vi "24C and 4G Read (SubVI).vi"(11 "Instrument":T4={"335 Resource"="", "Input (0:A)"=0, "Instrument Type"=enum."PPMS", "quantum design"=refnum, "Heater Output (1:1)"=0, "semaphore"=refnum, "TCP master instance"=refnum, "335 Status"=refnum, "M24C Resource"="GPIB0::24::INSTR", "4G supply"="GPIB0::24::INSTR", "Temp Status 24C"=refnum, "Temp"=refnum, "9T信号"=refnum, "limit"={"Field limit"=0.0, "Field rate limit"=0.0, "Temp limit"=0.0, "Temp low limit"=0.0, "Temp rate limit "=0.0}, "4g supply status"=refnum, "vi路径"=""} {"Input (0:A)" items=["A", "B"]; "Heater Output (1:1)" items=["1"=1, "2"=2]}) -> (0 "field status":T1=enum."Stable", 1 "field(Oe)":dbl, 2 "输出簇":T3 {"Loop1 Output (%)" format="%.2f"; "Loop2 Output (%)" format="%.2f"}, 3 "下拉列表":T2 items=["Unknow", "Stable", "Following Warm", "Following Cold", "Unfollowing"])   [LabVIEW 2019, in "9T cmag.lvlib"]
uses:
  9T cmag.lvlib
  ctl/Instrument.ctl
  <vilib>/NI/Modbus Library/API/Master/Modbus Master.lvclass
  ctl/Instrument Type.ctl
  lib/QDInstrument.dll
  ctl/335 state.ctl
  ctl/limit.ctl
  ctl/9T mag field stauts.ctl
  User lib.lvlib
panel:
  out "x-y 2":dbl
  out "x-y":dbl
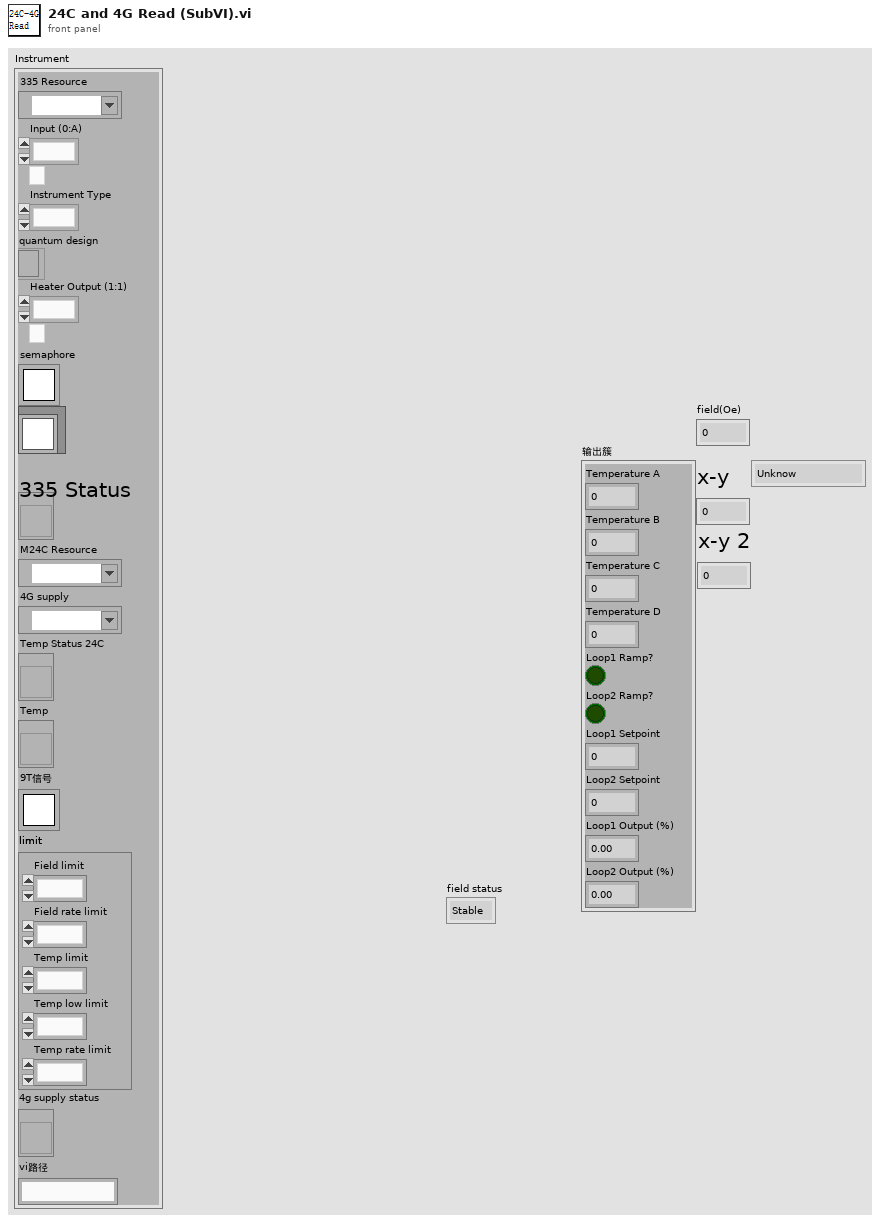
[diagram p1: front panel]
types:
  T1 = typedef "9T mag field stauts.ctl" = enum16{"unknow", "Stable", "Sweep up", "Sweep down", "Sweep to zero", "Pause"}
  T2 = typedef "335 state.ctl" = u16
  T3 = cluster{"Temperature A":dbl, "Temperature B":dbl, "Temperature C":dbl, "Temperature D":dbl, "Loop1 Ramp?":bool, "Loop2 Ramp?":bool, "Loop1 Setpoint":dbl, "Loop2 Setpoint":dbl, "Output Pwr (%)":dbl, "Output Pwr (%)":dbl}
  T4 = typedef "Instrument.ctl" = cluster{"335 Resource":refnum<visa-resource-name>, "Input (0:A)":u16, "Instrument Type":T5, "quantum design":refnum<k24>, "Heater Output (1:1)":u16, "semaphore":T6, "TCP master instance":refnum<class "Modbus Master.lvclass">, "335 Status":refnum<vi>, "M24C Resource":refnum<visa-resource-name>, "4G supply":refnum<visa-resource-name>, "Temp Status 24C":refnum<vi>, "Temp":refnum<vi>, "9T信号":T6, "limit":T7, "4g supply status":refnum<vi>, "vi路径":string}
  T5 = typedef "Instrument Type.ctl" = enum16{"PPMS", "VersaLab", "DynaCool", "SVSM", "PPMS-Rotate", "Lakeshore335", "9T mag"}
  T6 = typedef "Semaphore RefNum" = refnum<k1>
  T7 = typedef "limit.ctl" = cluster{"Field limit":dbl, "Field rate limit":dbl, "Temp limit":dbl, "Temp low limit":dbl, "Temp rate limit ":dbl}
  T8 = cluster{"Temperature":dbl, "Temperature":dbl, "Temperature":dbl, "Temperature":dbl, "x = y?":bool, "x = y?":bool, "数字":dbl, "数字":dbl, "Output Pwr (%)":dbl, "Output Pwr (%)":dbl}
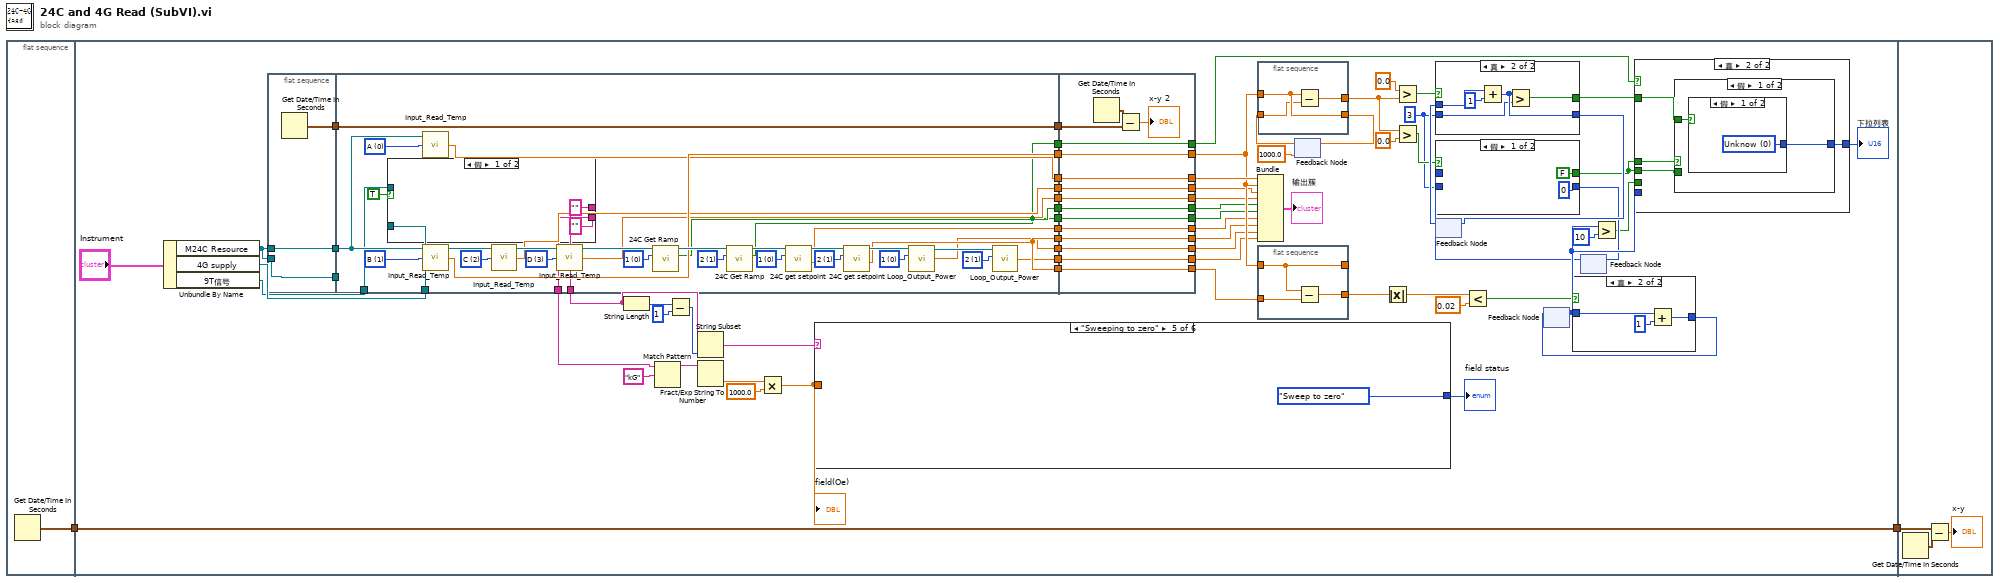
[diagram p0: block diagram]
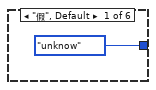
[diagram p2: hidden frame]
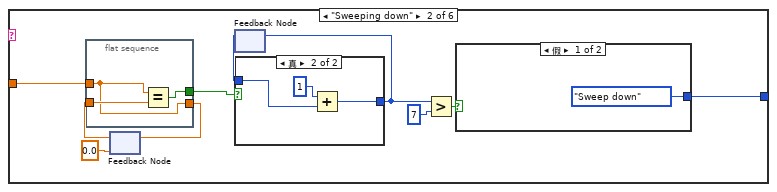
[diagram p3: hidden frame]
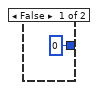
[diagram p4: hidden frame]
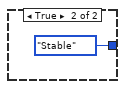
[diagram p5: hidden frame]
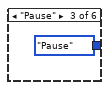
[diagram p6: hidden frame]
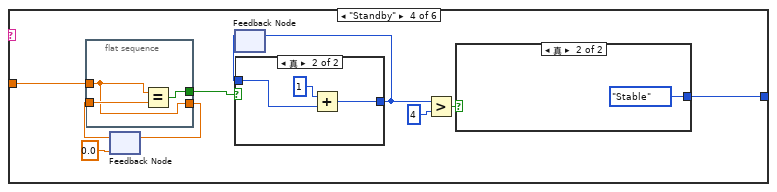
[diagram p7: hidden frame]
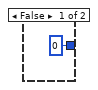
[diagram p8: hidden frame]
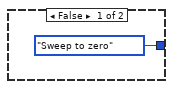
[diagram p9: hidden frame]
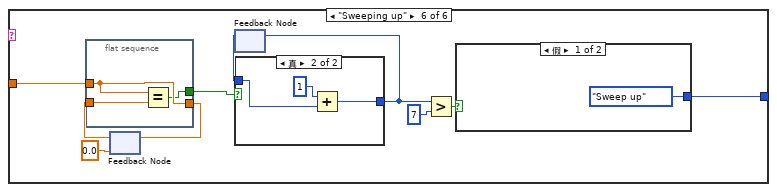
[diagram p10: hidden frame]
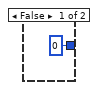
[diagram p11: hidden frame]
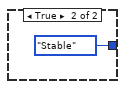
[diagram p12: hidden frame]
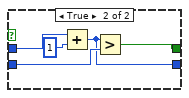
[diagram p13: hidden frame]
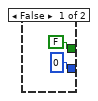
[diagram p14: hidden frame]
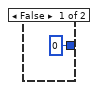
[diagram p15: hidden frame]
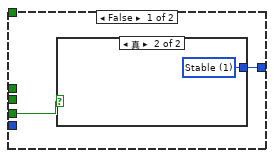
[diagram p16: hidden frame]
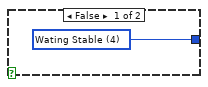
[diagram p17: hidden frame]
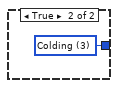
[diagram p18: hidden frame]
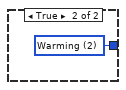
[diagram p19: hidden frame]
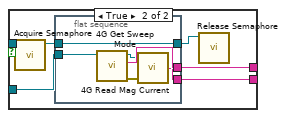
[diagram p20: hidden frame]
diagram:
  n1 = flat-sequence {
    tunnel: [w3] -> w2
    tunnel: w2 -> [w34]
    tunnel: [w34] -> w1
    tunnel: w1 -> [w240]
    frame #0 {
      n2 = Get Date/Time In Seconds() -> (seconds since 1Jan1904=w3:timestamp)
    }
    frame #1 {
      w57 = 3 ("y")
      n3 = Unbundle By Name("Instrument") -> ("M24C Resource"=w56:refnum<visa-resource-name>, "4G supply"=w35:refnum<visa-resource-name>, "9T信号"=w16:T6)
      n4 = flat-sequence {
        tunnel: w56 -> [w172]
        tunnel: w56 -> [w173]
        tunnel: [w173] -> w33
        tunnel: [w172] -> w32
        tunnel: [w171] -> w19
        tunnel: [w176] -> w4
        tunnel: [w180] -> w7
        tunnel: w35 -> [w179]
        tunnel: w33 -> [_]
        tunnel: w32 -> [w178]
        tunnel: [w195] -> w31
        tunnel: [w185] -> w30
        tunnel: [w183] -> w29
        tunnel: [w189] -> w28
        tunnel: [w188] -> w27
        tunnel: [w187] -> w26
        tunnel: [w186] -> w25
        tunnel: [w185] -> w24
        tunnel: [w184] -> w23
        tunnel: [w183] -> w22
        tunnel: [w182] -> w21
        tunnel: [w181] -> w20
        tunnel: w19 -> [w177]
        tunnel: [w177] -> w18
        tunnel: w16 -> [w175]
        tunnel: [w226] -> w37
        tunnel: [w227] -> w38
        tunnel: [w228] -> w39
        tunnel: [w229] -> w40
        tunnel: [w230] -> w41
        tunnel: [w231] -> w42
        tunnel: [w232] -> w43
        tunnel: [w233] -> w44
        tunnel: [w234] -> w46
        tunnel: [w235] -> w52
        tunnel: [w236] -> w53
        tunnel: [w237] -> w45
        tunnel: w31 -> [w237]
        tunnel: w30 -> [w236]
        tunnel: w29 -> [w235]
        tunnel: w28 -> [w234]
        tunnel: w27 -> [w233]
        tunnel: w26 -> [w232]
        tunnel: w25 -> [w231]
        tunnel: w24 -> [w230]
        tunnel: w23 -> [w229]
        tunnel: w22 -> [w228]
        tunnel: w21 -> [w227]
        tunnel: w20 -> [w226]
        tunnel: w18 -> [w224]
        frame #0 {
          n5 = Get Date/Time In Seconds() -> (seconds since 1Jan1904=w171:timestamp)
        }
        frame #1 {
          w191 = u8 1 items=["1", "2", "3", "4"] ("Loop")
          w193 = u8 0 items=["1", "2", "3", "4"] ("Loop")
          w196 = u8 1 items=["1", "2", "3", "4"] ("Loop")
          w197 = u8 0 items=["1", "2", "3", "4"] ("Loop")
          w199 = u8 1 items=["1", "2", "3", "4"] ("Loop")
          w201 = u8 0 items=["1", "2", "3", "4"] ("Loop")
          w203 = u8 3 items=["A", "B", "C", "D"] ("Input")
          w205 = u8 2 items=["A", "B", "C", "D"] ("Input")
          w207 = u8 1 items=["A", "B", "C", "D"] ("Input")
          w208 = u8 0 items=["A", "B", "C", "D"] ("Input")
          n6 = case shown="假" TRUE {
            tunnel: ["" ("response out") w216] -> w180
            tunnel: w179 -> [_ w215]
            tunnel: ["" ("response out") w214] -> w176
            tunnel: w175 -> [_ w212]
            frame False {
            }
            frame True {
              n7 = call <vilib>:"Acquire Semaphore.vi"("semaphore"=w212) -> ("semaphore out"=w213:T6)  [unwired: 4 in, 2 out]
              n8 = flat-sequence {
                tunnel: [w222] -> w216
                tunnel: w215 -> [w221]
                tunnel: [w220] -> w214
                tunnel: w213 -> [w218]
                tunnel: [w218] -> w211
                frame #0 {
                  n9 = call "4G Get Sweep Mode.vi"("VISA session"=w221) -> ("error out"=w217:errorcluster, "response out"=w222:string, "dup VISA session"=w219:refnum<visa-resource-name>)  [unwired: 3 in, 1 out]
                  n10 = call "4G Read Mag Current.vi"("error in (no error)"=w217, "VISA session"=w219) -> ("response out"=w220:string)  [unwired: 1 in, 2 out]
                }
              }
              n11 = call <vilib>:"Release Semaphore.vi"("semaphore"=w211) -> ()  [unwired: 5 in, 2 out]
            }
          }
          n12 = call "Input_Read_Temp.vi"("Input"=w208, "VISA In"=w178) -> ("Temperature"=w189:dbl)  [unwired: 1 in, 2 out]
          n13 = call "Input_Read_Temp.vi"("Input"=w207, "VISA In"=w178) -> ("Temperature"=w195:dbl, "VISA Out"=w206:refnum<visa-resource-name>)  [unwired: 1 in, 1 out]
          n14 = call "Input_Read_Temp.vi"("Input"=w205, "VISA In"=w206) -> ("Temperature"=w188:dbl, "VISA Out"=w204:refnum<visa-resource-name>)  [unwired: 1 in, 1 out]
          n15 = call "Input_Read_Temp.vi"("Input"=w203, "VISA In"=w204) -> ("Temperature"=w187:dbl, "VISA Out"=w202:refnum<visa-resource-name>)  [unwired: 1 in, 1 out]
          n16 = call "24C Get Ramp.vi"("Loop"=w201, "VISA in"=w202) -> ("x = y?"=w186:bool, "VISA out"=w200:refnum<visa-resource-name>)  [unwired: 7 in, 1 out]
          n17 = call "24C Get Ramp.vi"("Loop"=w199, "VISA in"=w200) -> ("x = y?"=w185:bool, "VISA out"=w194:refnum<visa-resource-name>)  [unwired: 7 in, 1 out]
          n18 = call "24C get setpoint.vi"("Loop"=w193, "VISA In"=w194) -> ("数字"=w184:dbl, "VISA out"=w192:refnum<visa-resource-name>)  [unwired: 6 in, 1 out]
          n19 = call "24C get setpoint.vi"("Loop"=w191, "VISA In"=w192) -> ("数字"=w183:dbl, "VISA out"=w190:refnum<visa-resource-name>)  [unwired: 6 in, 1 out]
          n20 = call "Loop_Output_Power.vi"("VISA in"=w190, "Loop"=w197) -> ("VISA out"=w198:refnum<visa-resource-name>, "Output Pwr (%)"=w182:dbl)  [unwired: 3 in, 1 out]
          n21 = call "Loop_Output_Power.vi"("VISA in"=w198, "Loop"=w196) -> ("Output Pwr (%)"=w181:dbl)  [unwired: 3 in, 2 out]
        }
        frame #2 {
          n22 = Get Date/Time In Seconds() -> (seconds since 1Jan1904=w225:timestamp)
          n23 = Subtract(x=w225, y=w224) -> (x-y=→"x-y 2":dbl)
        }
      }
      n24 = String Length(string=w7) -> (length=w8:i32)
      n25 = Match Pattern(string=w4, regular expression="kG" ("正则表达式")) -> (before substring=w14:string)  [unwired: 1 in, 3 out]
      n26 = Subtract(x=w8, y=1) -> (x-y=w9:i32)
      n27 = String Subset(string=w7, length (rest)=w9) -> (substring=w6:string)  [unwired: 1 in]
      n28 = Fract/Exp String To Number(string=w14) -> (number=w13:dbl)  [unwired: 3 in, 1 out]
      n29 = Multiply(x=w13, y=1000.0) -> (x*y=w5:dbl)
      "field(Oe)" <- w5
      n30 = case shown="\"Sweeping to zero\"" w6 {
        tunnel: [9T_mag_field_stauts."unknow" ("field stauts") w84 9T_mag_field_stauts."Pause" ("field stauts") w104 9T_mag_field_stauts."Sweep to zero" ("field stauts") w124] -> w11
        tunnel: w5 -> [_ w83 _ w103 _ w123]
        frame "假", Default {
        }
        frame "Sweeping down" {
          n31 = flat-sequence {
            tunnel: w83 -> [w90]
            tunnel: w81 -> [w91]
            tunnel: [w90] -> w82
            tunnel: [w89] -> w80
            frame #0 {
              n32 = Equal?(x=w90, y=w91) -> (x = y?=w89:bool)
            }
          }
          n33 = feedback-in #1(w82) -> ()
          n34 = feedback #1(0.0) -> (w81:dbl)
          n35 = feedback #2() -> (w79:i32)  [unwired: 1 in]
          n36 = case shown="真" w80 {
            tunnel: [0 w86] -> w78
            tunnel: w79 -> [_ w88]
            frame False {
            }
            frame True {
              n37 = Add(x=1, y=w88) -> (x+y=w86:i32)
            }
          }
          n38 = feedback-in #2(w78) -> ()
          n39 = Greater?(x=w78, y=7) -> (0:w76:bool)
          n40 = case shown="假" w76 {
            tunnel: [9T_mag_field_stauts."Sweep down" ("field stauts") 9T_mag_field_stauts."Stable" ("field stauts")] -> w84
            frame False {
            }
            frame True {
            }
          }
        }
        frame "Pause" {
        }
        frame "Standby" {
          n41 = flat-sequence {
            tunnel: w103 -> [w110]
            tunnel: w101 -> [w111]
            tunnel: [w110] -> w102
            tunnel: [w109] -> w100
            frame #0 {
              n42 = Equal?(x=w110, y=w111) -> (x = y?=w109:bool)
            }
          }
          n43 = feedback-in #3(w102) -> ()
          n44 = feedback #3(0.0) -> (w101:dbl)
          n45 = feedback #4() -> (w99:i32)  [unwired: 1 in]
          n46 = case shown="真" w100 {
            tunnel: [0 w106] -> w98
            tunnel: w99 -> [_ w108]
            frame False {
            }
            frame True {
              n47 = Add(x=1, y=w108) -> (x+y=w106:i32)
            }
          }
          n48 = feedback-in #4(w98) -> ()
          n49 = Greater?(x=w98, y=4) -> (0:w96:bool)
          n50 = case shown="真" w96 {
            tunnel: [9T_mag_field_stauts."Sweep to zero" ("field stauts") 9T_mag_field_stauts."Stable" ("field stauts")] -> w104
            frame False {
            }
            frame True {
            }
          }
        }
        frame "Sweeping to zero" {
        }
        frame "Sweeping up" {
          n51 = flat-sequence {
            tunnel: w123 -> [w130]
            tunnel: w121 -> [w131]
            tunnel: [w130] -> w122
            tunnel: [w129] -> w120
            frame #0 {
              n52 = Equal?(x=w130, y=w131) -> (x = y?=w129:bool)
            }
          }
          n53 = feedback-in #5(w122) -> ()
          n54 = feedback #5(0.0) -> (w121:dbl)
          n55 = feedback #6() -> (w119:i32)  [unwired: 1 in]
          n56 = case shown="真" w120 {
            tunnel: [0 w126] -> w118
            tunnel: w119 -> [_ w128]
            frame False {
            }
            frame True {
              n57 = Add(x=1, y=w128) -> (x+y=w126:i32)
            }
          }
          n58 = feedback-in #6(w118) -> ()
          n59 = Greater?(x=w118, y=7) -> (0:w116:bool)
          n60 = case shown="假" w116 {
            tunnel: [9T_mag_field_stauts."Sweep up" ("field stauts") 9T_mag_field_stauts."Stable" ("field stauts")] -> w124
            frame False {
            }
            frame True {
            }
          }
        }
      }
      "field status" <- w11
      n61 = flat-sequence {
        tunnel: w45 -> [w136]
        tunnel: [w136] -> w49
        tunnel: w51 -> [w135]
        tunnel: [w134] -> w50
        frame #0 {
          n62 = Subtract(x=w136, y=w135) -> (x-y=w134:dbl)
        }
      }
      n63 = Bundle("Temperature"=w46, "Temperature"=w45, "Temperature"=w44, "Temperature"=w43, "x = y?"=w42, "x = y?"=w41, "数字"=w40, "数字"=w39, "Output Pwr (%)"=w38, "Output Pwr (%)"=w37) -> (→"输出簇":T8)  [unwired: 1 in]
      n64 = flat-sequence {
        tunnel: w45 -> [w153]
        tunnel: [w153] -> _
        tunnel: w52 -> [w152]
        tunnel: [w151] -> w55
        frame #0 {
          n65 = Subtract(x=w153, y=w152) -> (x-y=w151:dbl)
        }
      }
      n66 = feedback #7(1000.0 ("Setpoint")) -> (w51:dbl)
      n67 = feedback-in #7(w49) -> ()
      n68 = Absolute Value(x=w55) -> (abs(x)=w67:dbl)
      n69 = Greater?(x=0.0, y=w50) -> (0:w63:bool)
      n70 = Greater?(x=w50, y=0.0) -> (0:w58:bool)
      n71 = feedback #8() -> (w61:i32)  [unwired: 1 in]
      n72 = case shown="真" w63 {
        tunnel: [0 w148] -> w62
        tunnel: w61 -> [_ w149]
        tunnel: w57 -> [_ w147]
        tunnel: [FALSE w146] -> w47
        frame False {
        }
        frame True {
          n73 = Add(x=w149, y=1) -> (x+y=w148:i32)
          n74 = Greater?(x=w148, y=w147) -> (0:w146:bool)
        }
      }
      n75 = feedback-in #8(w62) -> ()
      n76 = Less?(x=w67, y=0.02) -> (x < y?=w66:bool)
      n77 = feedback #9() -> (w70:i32)  [unwired: 1 in]
      n78 = case shown="真" w66 {
        tunnel: w70 -> [_ w157]
        tunnel: [0 w155] -> w69
        frame False {
        }
        frame True {
          n79 = Add(x=w157, y=1) -> (x+y=w155:i32)
        }
      }
      n80 = feedback-in #9(w69) -> ()
      n81 = feedback #10() -> (w60:i32)  [unwired: 1 in]
      n82 = case shown="假" w58 {
        tunnel: [0 w140] -> w59
        tunnel: w60 -> [_ w142]
        tunnel: w57 -> [_ w141]
        tunnel: [FALSE w139] -> w48
        frame False {
        }
        frame True {
          n83 = Add(x=w142, y=1) -> (x+y=w140:i32)
          n84 = Greater?(x=w140, y=w141) -> (0:w139:bool)
        }
      }
      n85 = feedback-in #10(w59) -> ()
      n86 = Greater?(x=w70, y=10) -> (0:w54:bool)
      n87 = case shown="真" w53 {
        tunnel: w70 -> [_ _]
        tunnel: w54 -> [w159 _]
        tunnel: [w158 w162] -> w17
        tunnel: w48 -> [_ w165]
        tunnel: w48 -> [_ w164]
        tunnel: w47 -> [_ w163]
        frame False {
          n88 = case shown="真" w159 {
            tunnel: [w160 w161] -> w158
            frame False {
              w160 = T2 4 items=["Unknow", "Stable", "Warming", "Colding", "Wating Stable"]
            }
            frame True {
              w161 = T2 1 items=["Unknow", "Stable", "Following Warm", "Following Cold", "Unfollowing"]
            }
          }
        }
        frame True {
          n89 = case shown="假" w164 {
            tunnel: w165 -> [_ _]
            tunnel: w163 -> [w167 _]
            tunnel: [w166 w170] -> w162
            frame False {
              n90 = case shown="假" w167 {
                tunnel: [w168 w169] -> w166
                frame False {
                  w168 = T2 0 items=["Unknow", "Stable", "Following Warm", "Following Cold", "Unfollowing"]
                }
                frame True {
                  w169 = T2 3 items=["Unknow", "Stable", "Warming", "Colding", "Wating Stable"]
                }
              }
            }
            frame True {
              w170 = T2 2 items=["Unknow", "Stable", "Warming", "Colding", "Wating Stable"]
            }
          }
        }
      }
      "下拉列表" <- w17
    }
    frame #2 {
      n91 = Get Date/Time In Seconds() -> (seconds since 1Jan1904=w239:timestamp)
      n92 = Subtract(x=w240, y=w239) -> (x-y=→"x-y":dbl)
    }
  }
